vi "Voltage_comparator.vi"(2 "Data":dbl[](array[numeric]), 3 "dt":dbl, 4 "V_Hysteris":dbl=0.03 format="%#_13g", 5 "V_thr":dbl) -> (0 "Waveform":waveform(i16), 1 "Pulse Dur":i32)   [LabVIEW 2015]
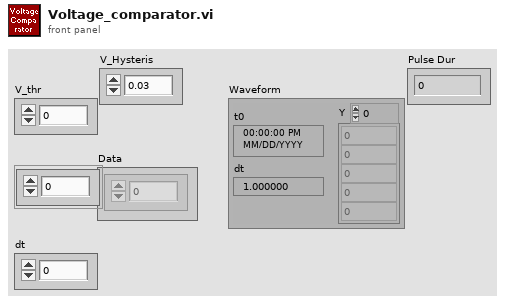
[diagram p1: front panel]
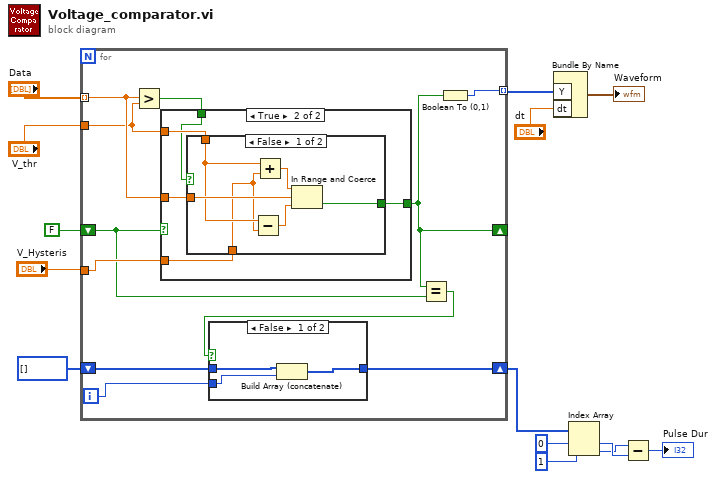
[diagram p0: block diagram]
diagram:
  n1 = for {
    tunnel: "Data" -> [w24] mode=indexing
    tunnel: [w25] -> w10 mode=indexing
    shift-right: [w20] -> _
    shift-left: FALSE -> [w19]
    tunnel: "V_thr" -> [w22]
    tunnel: "V_Hysteris" -> [w21]
    shift-right: [w16] -> w6
    shift-left: i32[] [] ("appended array") -> [w17]
    i -> [w15]
    n2 = Greater?(x=w24, y=w22) -> (0:w23:bool)
    n3 = case shown="True" w19 {
      tunnel: w24 -> [_ w35]
      tunnel: w22 -> [_ w34]
      tunnel: [w30 w33] -> w20
      tunnel: w23 -> [w30 w32]
      tunnel: w21 -> [_ w31]
      frame False {
      }
      frame True {
        n4 = case shown="False" w32 {
          selector: w32 -> [_ w42]
          tunnel: w35 -> [w41 _]
          tunnel: w34 -> [w39 _]
          tunnel: [w37 w42] -> w33
          tunnel: w31 -> [w36 _]
          frame False {
            n5 = Subtract(x=w39, y=w36) -> (x-y=w38:dbl)
            n6 = Add(x=w39, y=w36) -> (x+y=w40:dbl)
            n7 = In Range and Coerce(upper limit=w40, x=w41, lower limit=w38) -> (In Range?=w37:bool)  [unwired: 1 out]
          }
          frame True {
          }
        }
      }
    }
    n8 = Equal?(x=w20, y=w19) -> (x = y?=w18:bool)
    n9 = case shown="False" w18 {
      tunnel: [w27 w29] -> w16
      tunnel: w17 -> [w28 w29]
      tunnel: w15 -> [w26 _]
      frame False {
        n10 = Build Array (concatenate)(w28, w26) -> (w27:i32[])
      }
      frame True {
      }
    }
    n11 = Boolean To (0,1)(Boolean=w20) -> (0, 1=w25:i16)
  }
  n12 = Bundle By Name("Y"=w10, "dt"="dt") -> (→"Waveform":waveform(i16))  [unwired: 1 in]
  n13 = Index Array(array=w6, index #1=0 ("index"), index #2=1 ("index")) -> (element #1=w3:i32, element #2=w2:i32)
  n14 = Subtract(x=w2, y=w3) -> (x-y=→"Pulse Dur":i32)
